vi "ex14-8.vi"(1 "數值":dbl) -> (0 "溢位?":bool)   [LabVIEW 2014]
uses:
  <vilib>/NXT/Subs/MotorOutput.ctl
  <vilib>/NXT/Dual Mode Library/Motors/MotorDistance_Single.vi
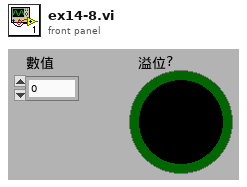
[diagram p1: front panel]
types:
  T1 = typedef "MotorOutput.ctl" = u8
  T2 = typedef "LVHSConnector.ctl" = refnum<class "BrickReference.lvclass">
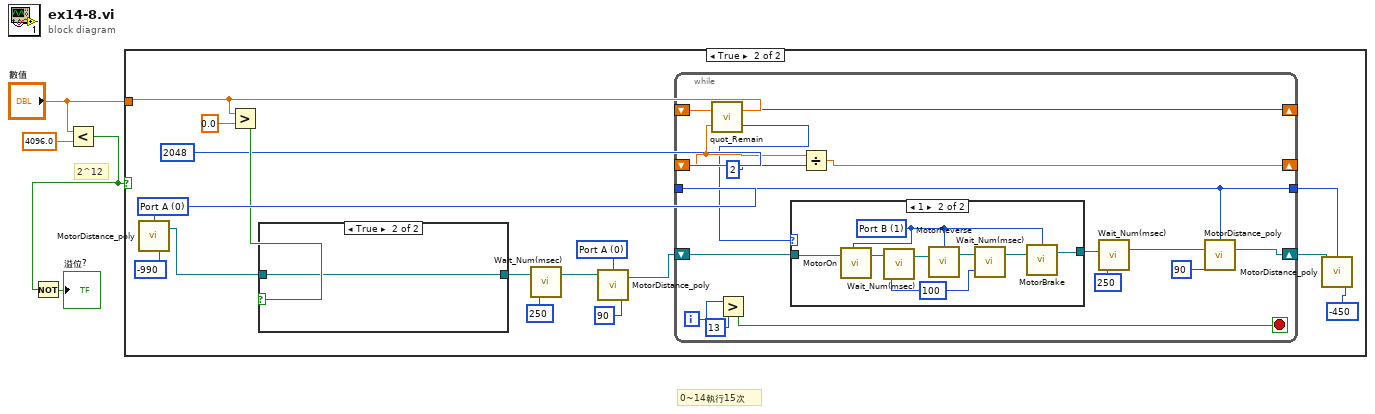
[diagram p0: block diagram]
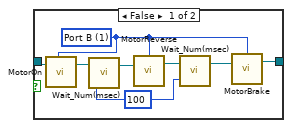
[diagram p3: hidden frame]
diagram:
  # "0~14執行15次"
  # "2^12"
  n1 = Less?(x="數值", y=4096.0) -> (x < y?=w4:bool)
  n2 = Not(x=w4) -> (.not. x?=→"溢位?":bool)
  n3 = case shown="True" w4 {
    tunnel: "數值" -> [_ w6]
    frame False {
    }
    frame True {
      w7 = T1 0 items=["Port A", "Port B", "Port C", "All Ports"] ("Output Port (All Ports)")
      w17 = T1 0 items=["Port A", "Port B", "Port C", "All Ports"] ("Output Port (All Ports)")
      n4 = call-poly <vilib>:"MotorDistance_poly.vi"("Angle of Rotation (360)"=-990 ("Distance (100)"), "Output Port (All Ports)"=w17) -> ("NXT/EV3"=w13:T2)  [unwired: 2 in]
      n5 = Greater?(x=w6, y=0.0) -> (0:w14:bool)
      n6 = case shown="True" w14 {
        tunnel: w13 -> [w21 w29]
        tunnel: [w22 w29] -> w8
        frame False {
          w28 = u32 100 ("Time (100 msec)")
          w23 = T1 1 items=["Port A", "Port B", "Port C", "All Ports"] ("Output Port (All Ports)")
          n7 = call <vilib>:"MotorOn.vi"("NXT/EV3"=w21, "Output Port (All Ports)"=w23) -> ("NXT/EV3"=w27:T2)  [unwired: 2 in]
          n8 = call <vilib>:"Wait_Num(msec).vi"("Time (100 msec)"=w28, "NXT/EV3"=w27) -> ("NXT/EV3"=w26:T2)  [unwired: 2 in]
          n9 = call <vilib>:"MotorReverse.vi"("NXT/EV3"=w26, "Output Port (All Ports)"=w23) -> ("NXT/EV3"=w25:T2)  [unwired: 2 in]
          n10 = call <vilib>:"Wait_Num(msec).vi"("Time (100 msec)"=w28, "NXT/EV3"=w25) -> ("NXT/EV3"=w24:T2)  [unwired: 2 in]
          n11 = call <vilib>:"MotorBrake.vi"("NXT/EV3"=w24, "Port (All Ports)"=w23) -> ("NXT/EV3"=w22:T2)  [unwired: 2 in]
        }
        frame True {
        }
      }
      n12 = call <vilib>:"Wait_Num(msec).vi"("Time (100 msec)"=u32 250, "NXT/EV3"=w8) -> ("NXT/EV3"=w10:T2)  [unwired: 2 in]
      n13 = call-poly <vilib>:"MotorDistance_poly.vi"("Angle of Rotation (360)"=90 ("Distance (100)"), "NXT/EV3"=w10, "Output Port (All Ports)"=w7) -> ("NXT/EV3"=w5:T2)  [unwired: 1 in]
      n14 = while {
        shift-right: [w31] -> _
        shift-left: w6 -> [w33]
        shift-right: [w44] -> _
        shift-left: 2048 -> [w32]
        shift-right: [w37] -> w19
        shift-left: w5 -> [w43]
        tunnel: w17 -> [w38]
        tunnel: [w38] -> w16
        i -> [w42]
        stop <- w40 stop-if-true
        n15 = call <vilib>:"quot_Remain.vi"("y"=w32, "x"=w33) -> ("floor(x/y)"=w30:i32, "x-y*floor(x/y)"=w31:i32)
        n16 = Greater?(x=w42, y=13) -> (0:w40:bool)
        n17 = case shown="1" w30 {
          tunnel: w43 -> [w46 w48]
          tunnel: [w46 w47] -> w36
          frame 0, Default {
          }
          frame 1 {
            w49 = u32 100 ("Time (100 msec)")
            w54 = T1 1 items=["Port A", "Port B", "Port C", "All Ports"] ("Output Port (All Ports)")
            n18 = call <vilib>:"MotorOn.vi"("NXT/EV3"=w48, "Output Port (All Ports)"=w54) -> ("NXT/EV3"=w50:T2)  [unwired: 2 in]
            n19 = call <vilib>:"Wait_Num(msec).vi"("Time (100 msec)"=w49, "NXT/EV3"=w50) -> ("NXT/EV3"=w51:T2)  [unwired: 2 in]
            n20 = call <vilib>:"MotorReverse.vi"("NXT/EV3"=w51, "Output Port (All Ports)"=w54) -> ("NXT/EV3"=w52:T2)  [unwired: 2 in]
            n21 = call <vilib>:"Wait_Num(msec).vi"("Time (100 msec)"=w49, "NXT/EV3"=w52) -> ("NXT/EV3"=w53:T2)  [unwired: 2 in]
            n22 = call <vilib>:"MotorBrake.vi"("NXT/EV3"=w53, "Port (All Ports)"=w54) -> ("NXT/EV3"=w47:T2)  [unwired: 2 in]
          }
        }
        n23 = Divide(x=w32, y=2) -> (x/y=w44:dbl)
        n24 = call <vilib>:"Wait_Num(msec).vi"("Time (100 msec)"=u32 250, "NXT/EV3"=w36) -> ("NXT/EV3"=w35:T2)  [unwired: 2 in]
        n25 = call-poly <vilib>:"MotorDistance_poly.vi"("Angle of Rotation (360)"=90 ("Distance (100)"), "NXT/EV3"=w35, "Output Port (All Ports)"=w38) -> ("NXT/EV3"=w37:T2)  [unwired: 1 in]
      }
      n26 = call-poly <vilib>:"MotorDistance_poly.vi"("Angle of Rotation (360)"=-450 ("Distance (100)"), "NXT/EV3"=w19, "Output Port (All Ports)"=w16) -> ()  [unwired: 1 in, 1 out]
    }
  }
